vi "Python_LabVIEW.vi"() -> ()   [LabVIEW 2026]
panel:
  in  "User input 3":dbl=3.0 format="%#_13g"
  in  "name or relative path":path=path "C:/GitHub_Repositories/LabVIEW_Python_Code_Runner/Python_LabVIEW.py"
  out "appended path":path=path "C:/Users/dernoczig/Desktop/_Phyton_Pycharm_Projects/Python_LabVIEW.py"
  out "return value":dbl
  in  "User input 2":dbl=3.0 format="%#_13g"
  in  "User input1":dbl=2.0 format="%#_13g"
  in  "Function name":string="LabVIEW"
  in  "Python version":string="3.12.0"
  # "C:\\Users\\derno\\AppData\\Local\\Programs\\Python\\Python312-32\\python.exe"
  # "output = 0\n\ndef LabVIEW(Input1, Input2, Input3):\n    output = Input1 + Input2 + Input3\n    print(output)\n    return (output)\n\n#LabVIEW(1,3,5)"
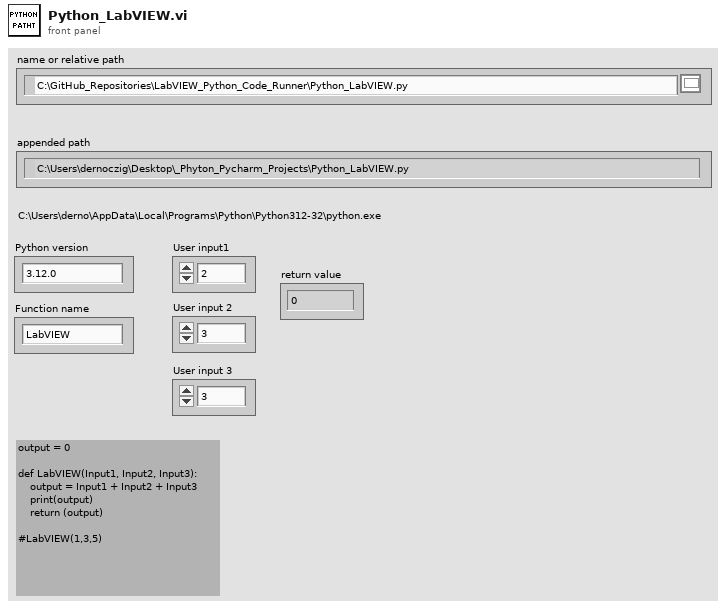
[diagram p1: front panel]
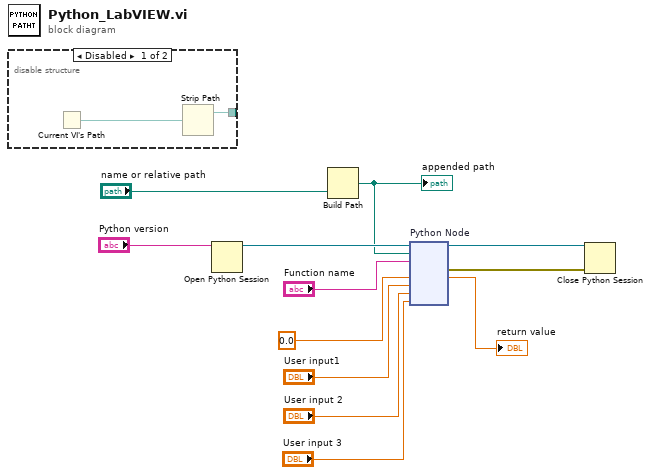
[diagram p0: block diagram]
diagram:
  n1 = disable-structure shown="Disabled" {
    disable-tunnel: [w13 _] -> _
    frame Disabled {
      n2 = Current VI's Path() -> (path=w14:path)
      n3 = Strip Path(path=w14) -> (stripped path=w13:path)  [unwired: 1 out]
    }
    frame Enabled {
    }
  }
  n4 = Open Python Session(python version="Python version") -> (session out=w11:refnum<k35>)  [unwired: 2 in, 1 out]
  n5 = Build Path(name or relative path="name or relative path") -> (appended path=w2:path)  [unwired: 1 in]
  "appended path" <- w2
  n6 = node "Python Node"(w11, w2, "Function name", 0.0, "User input1", "User input 2", "User input 3") -> (w5:refnum<k35>, w6:errorcluster, →"return value":dbl)  [unwired: 4 in, 2 out]
  n7 = Close Python Session(session in=w5, error in=w6) -> ()  [unwired: 1 out]
